vi "BaseDeviseBaseVI.vi"(8 "ErrorIn(No Error)":errorcluster caption="entrée d'erreur (pas d'erreur)", 11 "BaseDevice.lvclass":refnum<class "BaseDevice.lvclass">) -> (0 "sortie d'erreur":errorcluster, 3 "BaseDevice.lvclass Out":refnum<class "BaseDevice.lvclass">)   [LabVIEW 2019, in "BaseDevice.lvclass"]
uses:
  BaseDevice.lvclass
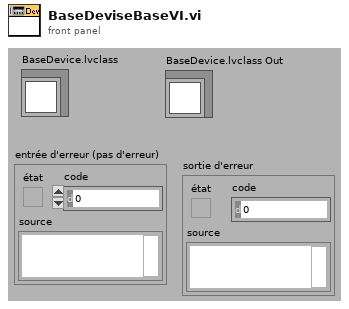
[diagram p1: front panel]
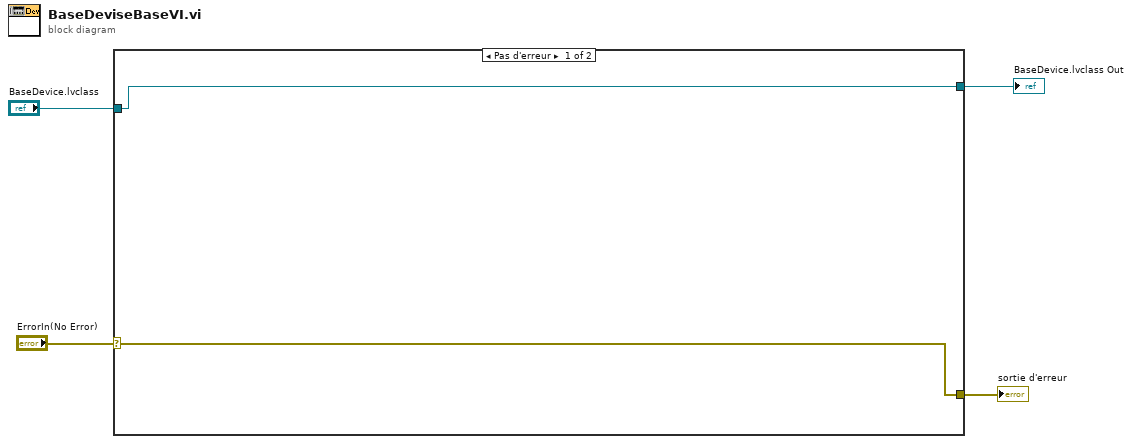
[diagram p0: block diagram]
diagram:
  n1 = case shown="Pas d'erreur" "ErrorIn(No Error)" {
    selector: "ErrorIn(No Error)" -> [w6 w8]
    tunnel: [w6 w8] -> w4
    tunnel: "BaseDevice.lvclass" -> [w5 w7]
    tunnel: [w5 w7] -> w1
    frame No Error {
    }
    frame Error {
    }
  }
  "sortie d'erreur" <- w4
  "BaseDevice.lvclass Out" <- w1
